vi "LINX - AD9850.vi"() -> ()   [LabVIEW 2011, in "LMH-LINX.lvlib"]
doc: "Set the output frequency and phase offset of a AD9850 DDS."
uses:
  vi.lib/MakerHub/LINX/LMH-LINX.lvlib
  vi.lib/MakerHub/LINX/Public/Sensors/Signal Generation/AD9850/AD9850.lvlib
panel:
  in  "Frequency":u32
  in  "Phase Offset (5-bit)":u8
  in  "Ref Clock Freq (125MHz)":dbl=125000000.0 format="%#_6p"
  in  "SPI Channel (0)":u8
  in  "CS Channel":u8
  out "Loop Rate (Hz)":u32
  in  "Serial Port":refnum<visa-resource-name>
  in  "Stop Button":bool
  # "AD9850 Control"
  # "Circuit Schematic"
  # "LINX Device Settings"
  # "AD9850 Configuration"
  # "AD9850 Example\n\nThis example demonstrates how to set output frequency and phase offset of an AD9850 DDS.\n\nNote: This example is configured to use a serial interface but can easily be modified\nto use TCP or run on myRIO.\n\nInstructions\n1. Select the COM Port associated with the LINX Device.\n2. Select the SPI Channel, CS Channel, and Ref Clock Frequency.\n3. Click the Run Arrow.\n4. Adjust the Frequency, and Phase."
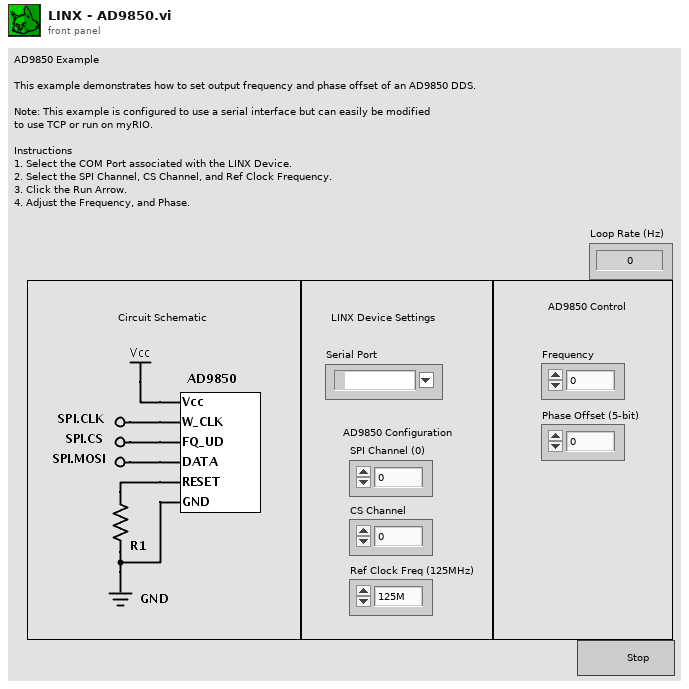
[diagram p1: front panel]
types:
  T1 = typedef "LMH-LINX.lvlib/LINX Ref.ctl" = cluster{"Platform":T2, "Interface":T3, "LINX Device Config":T4}
  T2 = typedef "LMH-LINX.lvlib/Platform.ctl" = enum16{"LINX", "myRIO"}
  T3 = typedef "LMH-LINX.lvlib/Interface.ctl" = enum16{"Serial", "TCP"}
  T4 = typedef "LMH-LINX.lvlib/Device.lvlib/LINX Device Config.ctl" = cluster{"Interface":T3, "COM Port":refnum<visa-resource-name>, "TCP Configuration":T5, "Device Family":u8, "Device ID":u8, "Device Name":string, "TCP Ref":refnum<k5>, "Channels":T6}
  T5 = typedef "LMH-LINX.lvlib/Device.lvlib/TCP Config.ctl" = cluster{"IP Address":string, "Port":u16}
  T6 = typedef "LMH-LINX.lvlib/Channels.ctl" = cluster{"DI":u8[], "DO":u8[], "AI":u8[], "AO":u8[], "PWM":u8[], "QE":u8[], "UART":u8[], "I2C 2":u8[], "SPI":u8[], "CAN":u8[], "Servo":u8[], "AI Ref (V)":dbl, "AO Ref (V)":dbl, "AO Resolution (Bits)":u8}
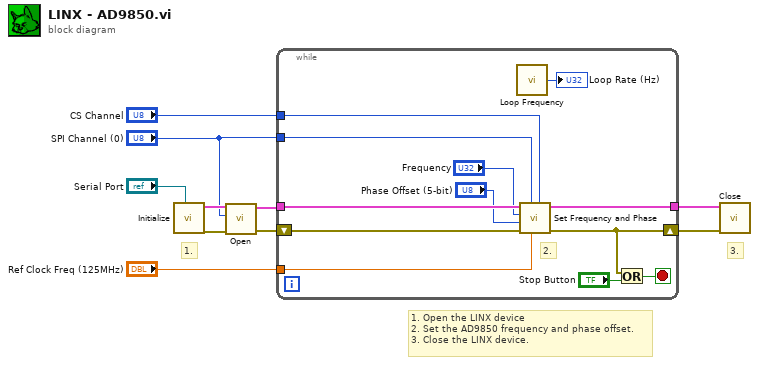
[diagram p0: block diagram]
diagram:
  # "3."
  # "1."
  # "1. Open the LINX device\n2. Set the AD9850 frequency and phase offset.\n3. Close the LINX device."
  n1 = call "Initialize.vi"("Serial Port"="Serial Port") -> ("Error Out"=w4:errorcluster, "LINX Ref"=w7:T1)  [unwired: 8 in, 1 out]
  n2 = call "Open.vi"("Error In"=w4, "SPI Channel (0)"="SPI Channel (0)", "LINX Resource"=w7) -> ("Error Out"=w5:errorcluster, "LINX Resource"=w6:T1)  [unwired: 7 in]
  n3 = while {
    shift-right: [w18] -> w10
    shift-left: w5 -> [w17]
    tunnel: [w12] -> w8
    tunnel: w6 -> [w19]
    tunnel: "Ref Clock Freq (125MHz)" -> [w16]
    tunnel: "SPI Channel (0)" -> [w15]
    tunnel: "CS Channel" -> [w11]
    stop <- w22 stop-if-true
    # "2."
    n4 = call "Loop Frequency.vi"() -> ("Loop Rate (Hz)"=→"Loop Rate (Hz)":u32)
    n5 = call "Set Frequency and Phase.vi"("CS Channel"=w11, "Ref Clock Freq (125MHz)"=w16, "SPI Channel (0)"=w15, "Error In"=w17, "Phase Offset (5-bit)"="Phase Offset (5-bit)", "Frequency"="Frequency", "LINX Resource"=w19) -> ("Error Out"=w18:errorcluster, "LINX Resource"=w12:T1)  [unwired: 3 in]
    n6 = Or(x=w18, y="Stop Button") -> (x .or. y?=w22:bool)
  }
  n7 = call "Close.vi"("Error In"=w10, "LINX Resource"=w8) -> ()  [unwired: 8 in, 2 out]
